vi "Connect.vi"(8 "error in (no error)":errorcluster, 10 "Partner URL":string, 11 "Network Stream Writer in":refnum<class "Network Stream Writer.lvclass">) -> (0 "error out":errorcluster, 3 "Network Stream Writer out":refnum<class "Network Stream Writer.lvclass">)   [LabVIEW 2014, in "Network Stream Writer.lvlib" / "Network Stream Writer.lvclass"]
uses:
  Network Stream Writer.lvclass
  Network Stream Writer.lvclass/Network Stream Writer.ctl
  Network Stream/Network Stream/MessageString.ctl
  <vilib>/ActorFramework/Message Enqueuer/Message Priority.ctl
  Network Stream/Network Stream/Network Stream.lvclass/Network Stream.ctl
  Proxy/Proxy/Proxy.lvclass/Proxy.ctl
  <vilib>/ActorFramework/Actor/Actor.lvclass/Actor.ctl
  Proxy/Proxy Messages/Proxy Status Msg/Proxy Status Msg.lvclass/Proxy Status Msg.ctl
  Network Stream/Network Stream/Read timeout.vi
  Network Stream/Network Stream/Read Buffer Size.vi
  Network Stream/Network Stream/Read Context.vi
  Network Stream/Network Stream/Read Name.vi
  Proxy/Proxy/Read Status Msg.vi
  Proxy/Proxy/Read Target Enq.vi
  <vilib>/ActorFramework/Message Enqueuer/Equals Not A Refnum.vi
  <vilib>/ActorFramework/Actor/Read Caller Enqueuer.vi
  Proxy/Proxy Messages/Proxy Status Msg/Proxy Status Msg.lvclass
  <vilib>/ActorFramework/Message Enqueuer/Message Enqueuer.lvclass
  Network Stream/Network Stream/Network Stream.lvclass
  <resource>/objmgr/ni.dex.rc
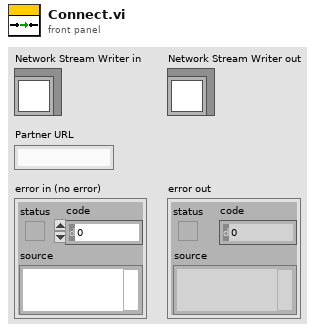
[diagram p1: front panel]
types:
  T1 = typedef "Network Stream.lvlib/Network Stream.lvclass/MessageString.ctl" = cluster{"Flatten Msg":string, "Message Priority":T2}
  T2 = typedef "Actor Framework.lvlib/Message Enqueuer.lvclass/Message Priority.ctl" = enum16{"Low", "Normal", "High"}
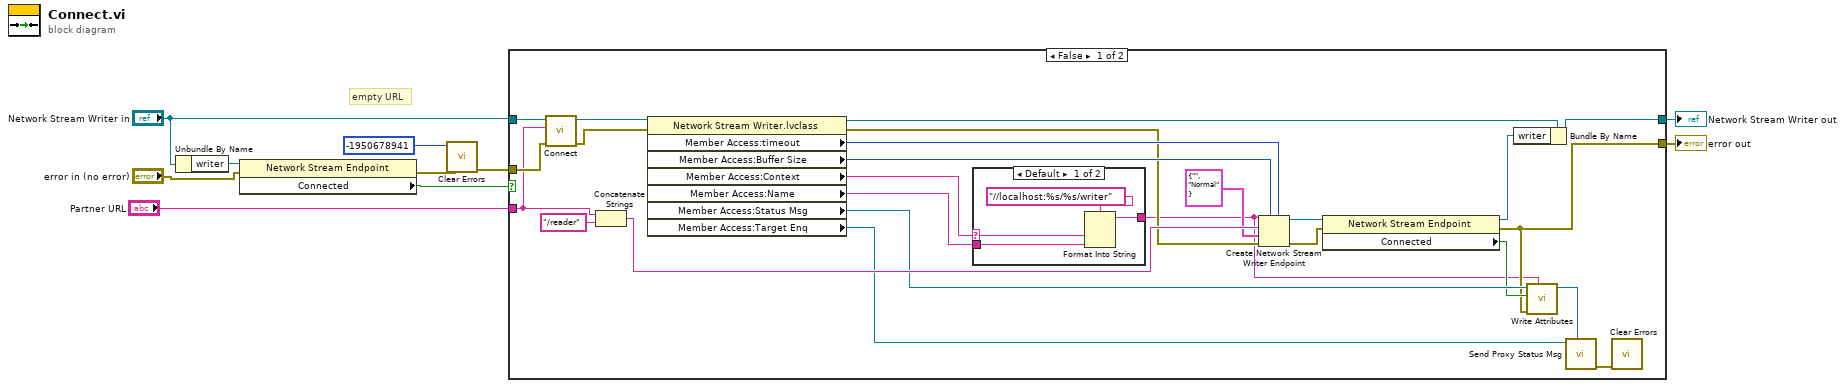
[diagram p0: block diagram]
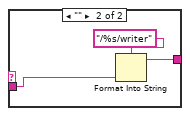
[diagram p2: hidden frame]
diagram:
  # "empty URL"
  n1 = Unbundle By Name("Network Stream Writer in") -> ("writer"=w6:refnum<k21>)
  n2 = property class="Network Stream Endpoint"(reference=w6, error in="error in (no error)") -> (error out=w3:errorcluster, "Connected"=w5:bool)  [unwired: 1 out]
  n3 = call <vilib>:"Clear Errors.vi"("error in (no error)"=w3, "specific error code to clear (0: all)"=-1950678941) -> ("error out"=w2:errorcluster)  [unwired: 4 in, 1 out]
  n4 = case shown="False" w5 {
    tunnel: w2 -> [w34 w44]
    tunnel: "Partner URL" -> [w30 _]
    tunnel: [w14 w44] -> w9
    tunnel: [w23 w43] -> w8
    tunnel: "Network Stream Writer in" -> [w20 w43]
    frame False {
      n5 = call-parent "Connect.vi"("error in (no error)"=w34, "Partner URL"=w30, "Proxy in"=w20) -> ("error out"=w25:errorcluster, "Proxy out"=w35:refnum<class "Network Stream Writer.lvclass">)  [unwired: 7 in]
      n6 = Concatenate Strings(w30, "/reader" ("string")) -> (w29:string)
      n7 = property class="Network Stream Writer.lvclass"(reference=w35, error in=w25) -> (reference out=w33:refnum<class "Network Stream Writer.lvclass">, error out=w24:errorcluster, "Member Access:timeout"=w31:i32, "Member Access:Buffer Size"=w32:i32, "Member Access:Context"=w27:string, "Member Access:Name"=w26:string, "Member Access:Status Msg"=w16:refnum<class "Proxy Status Msg.lvclass">, "Member Access:Target Enq"=w17:refnum<class "Message Enqueuer.lvclass">)
      n8 = case shown="Default" w27 {
        selector: w27 -> [w37 _]
        tunnel: [w38 w42] -> w12
        tunnel: w26 -> [w36 w40]
        frame Default {
          n9 = Format Into String(format string="//localhost:%s/%s/writer", w37, w36) -> (resulting string=w38:string)  [unwired: 2 in, 1 out]
        }
        frame "" {
          n10 = Format Into String(format string="/%s/writer", w40) -> (resulting string=w42:string)  [unwired: 2 in, 1 out]
        }
      }
      n11 = Create Network Stream Writer Endpoint(5:w31, 7:w32, 8:w24, 9:T1 {"Flatten Msg"="", "Message Priority"=enum."Normal"} ("Msg String"), 10:w29, 11:w12) -> (0:w18:errorcluster, 3:w22:refnum<k21>)  [unwired: 1 in]
      n12 = property class="Network Stream Endpoint"(reference=w22, error in=w18) -> (reference out=w19:refnum<k21>, error out=w14:errorcluster, "Connected"=w15:bool)
      n13 = Bundle By Name(cluster=w33, "writer"=w19) -> (w23:refnum<class "Network Stream Writer.lvclass">)
      n14 = call "Write Attributes.vi"("Name"=w12, "error in"=w14, "Writer"=w15, "Proxy Status Msg in"=w16) -> ("Proxy Status Msg out"=w13:refnum<class "Proxy Status Msg.lvclass">)  [unwired: 7 in]
      n15 = call "Send Proxy Status Msg.vi"("Message Type"=w13, "Message Enqueuer"=w17) -> ("error out"=w11:errorcluster)  [unwired: 8 in, 1 out]
      n16 = call <vilib>:"Clear Errors.vi"("error in (no error)"=w11) -> ()  [unwired: 5 in, 2 out]
    }
    frame True {
    }
  }
  "error out" <- w9
  "Network Stream Writer out" <- w8
